vi "Write ROI Descriptor.vi"(8 "error in (no error)":errorcluster, 10 "ROI Descriptor":T1, 11 "Video File in":refnum<class "Video File.lvclass">) -> (0 "error out":errorcluster, 3 "Video File out":refnum<class "Video File.lvclass">)   [LabVIEW 2018, in "Video File.lvclass"]
uses:
  Video File.lvclass
  Video File.lvclass/Video File.ctl
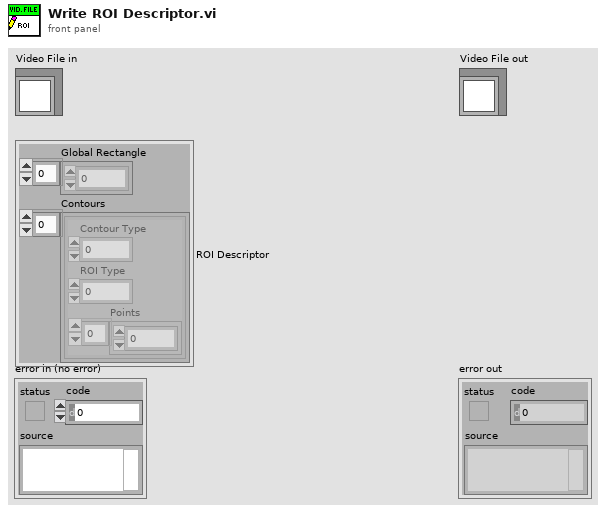
[diagram p1: front panel]
types:
  T1 = cluster{"Global Rectangle":i32[], "Contours":cluster{"Contour Type":u32, "ROI Type":u32, "Points":i32[]}[]}
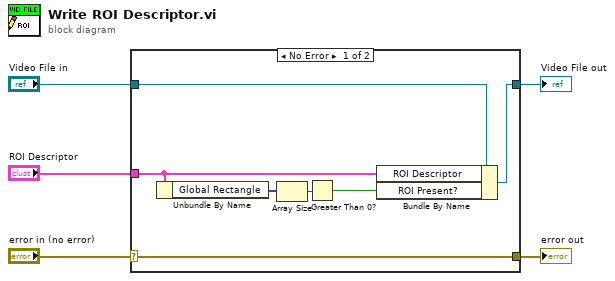
[diagram p0: block diagram]
diagram:
  n1 = case shown="No Error" "error in (no error)" {
    selector: "error in (no error)" -> [w12 w13]
    tunnel: [w12 w13] -> w4
    tunnel: [w10 w14] -> w2
    tunnel: "Video File in" -> [w11 w14]
    tunnel: "ROI Descriptor" -> [w9 _]
    frame No Error {
      n2 = Unbundle By Name(w9) -> ("Global Rectangle"=w8:i32[])
      n3 = Array Size(array=w8) -> (size(s)=w7:i32)
      n4 = Greater Than 0?(x=w7) -> (x > 0?=w6:bool)
      n5 = Bundle By Name(cluster=w11, "ROI Descriptor"=w9, "ROI Present?"=w6) -> (w10:refnum<class "Video File.lvclass">)
    }
    frame Error {
    }
  }
  "error out" <- w4
  "Video File out" <- w2
